vi "_f_BronkhorstExtract_SPPV.vi"(8 "error in (no error)":errorcluster, 10 "Read String":string) -> (0 "error out":errorcluster, 1 "Reading":T1, 2 "Setpoint":string)   [LabVIEW 2013]
panel:
  out "Command":string
  out "Param":string
  out "Process":string
  out "Node":string
  out "Lenght":string
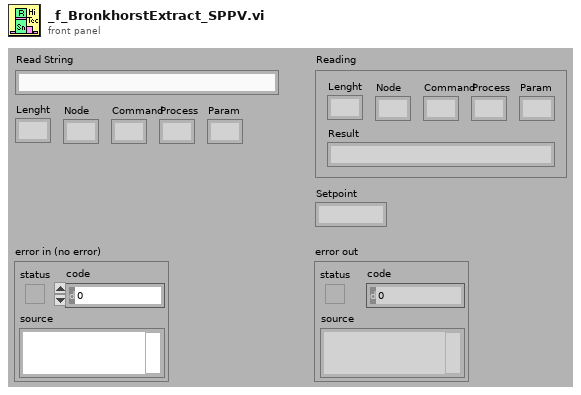
[diagram p1: front panel]
types:
  T1 = cluster{"Lenght":string, "Node":string, "Process":string, "Param":string, "Command":string, "Result":string}
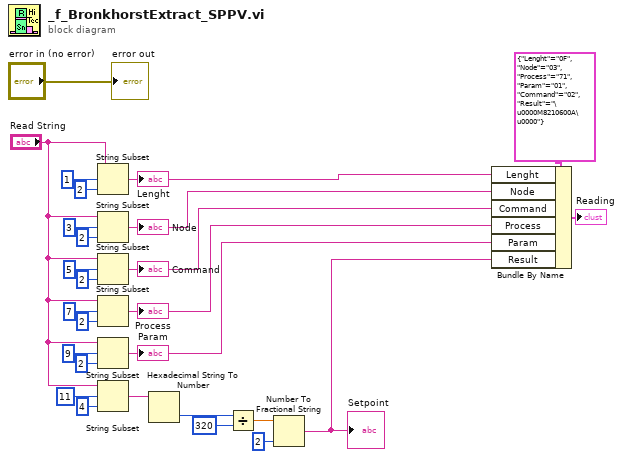
[diagram p0: block diagram]
diagram:
  n1 = String Subset(string="Read String", offset (0)=1, length (rest)=2 ("length (rest)")) -> (substring=w14:string)
  "Lenght" <- w14
  n2 = String Subset(string="Read String", offset (0)=3, length (rest)=2 ("length (rest)")) -> (substring=w13:string)
  "Node" <- w13
  n3 = String Subset(string="Read String", offset (0)=5, length (rest)=2 ("length (rest)")) -> (substring=w12:string)
  "Command" <- w12
  n4 = String Subset(string="Read String", offset (0)=7, length (rest)=2 ("length (rest)")) -> (substring=w11:string)
  "Process" <- w11
  n5 = String Subset(string="Read String", offset (0)=9, length (rest)=2 ("length (rest)")) -> (substring=w10:string)
  "Param" <- w10
  n6 = String Subset(string="Read String", offset (0)=11, length (rest)=4 ("length (rest)")) -> (substring=w6:string)
  n7 = Hexadecimal String To Number(string=w6) -> (number=w4:u32)  [unwired: 2 in, 1 out]
  n8 = Divide(x=w4, y=u32 320) -> (x/y=w2:dbl)
  n9 = Number To Fractional String(number=w2, precision (6)=i16 2) -> (F-format string=w5:string)  [unwired: 2 in]
  "Setpoint" <- w5
  n10 = Bundle By Name(cluster=T1 {"Lenght"="0F", "Node"="03", "Process"="71", "Param"="01", "Command"="02", "Result"="\u0000M8210600A\u0000"} ("Reading"), "Lenght"=w14, "Node"=w13, "Command"=w12, "Process"=w11, "Param"=w10, "Result"=w5) -> (→"Reading":T1)
  "error out" <- "error in (no error)"
